vi "DecodeRobotsVSS.vi"(4 "time stamp":timestamp, 5 "offset":i32, 7 "error in (no error)":errorcluster, 8 "array w/ subset deleted in":u8[](array[numeric])) -> (0 "error out":errorcluster, 1 "array w/ subset deleted out":u8[](array[numeric]), 3 "Array":T1[](array[typedef]) {"height" format="%+4.3f"; "pixel_y" format="%+4.3f"; "pixel_x" format="%+4.3f"; "orientation" format="%+4.3f"; "y" format="%+4.3f"; "confidence" format="%4.3f"; "x" format="%+4.3f"})   [LabVIEW 2017]
uses:
  SSL Detection Robot.ctl
  <vilib>/Analysis/Matrix/Datatypes/RealMatrix.ctl
  <vilib>/Analysis/Matrix/NI_Matrix.lvlib
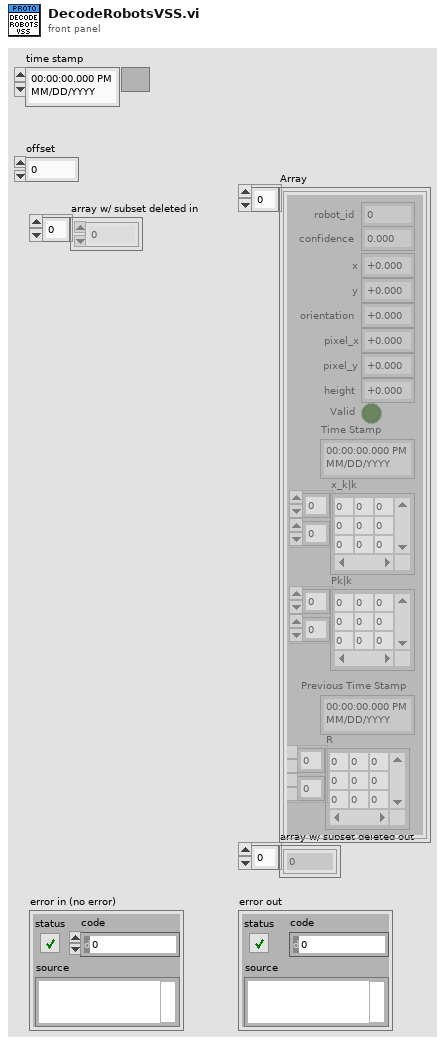
[diagram p1: front panel]
types:
  T1 = typedef "SSL Detection Robot.ctl" = cluster{"x":sgl, "robot_id":u32, "confidence":sgl, "y":sgl, "orientation":sgl, "pixel_x":sgl, "pixel_y":sgl, "height":sgl, "Valid":bool, "Time Stamp":timestamp, "x_k|k":T2, "Pk|k":T2, "Previous Time Stamp":timestamp, "R":T2}
  T2 = typedef "NI_Matrix.lvlib/RealMatrix.ctl" = dbl[][]
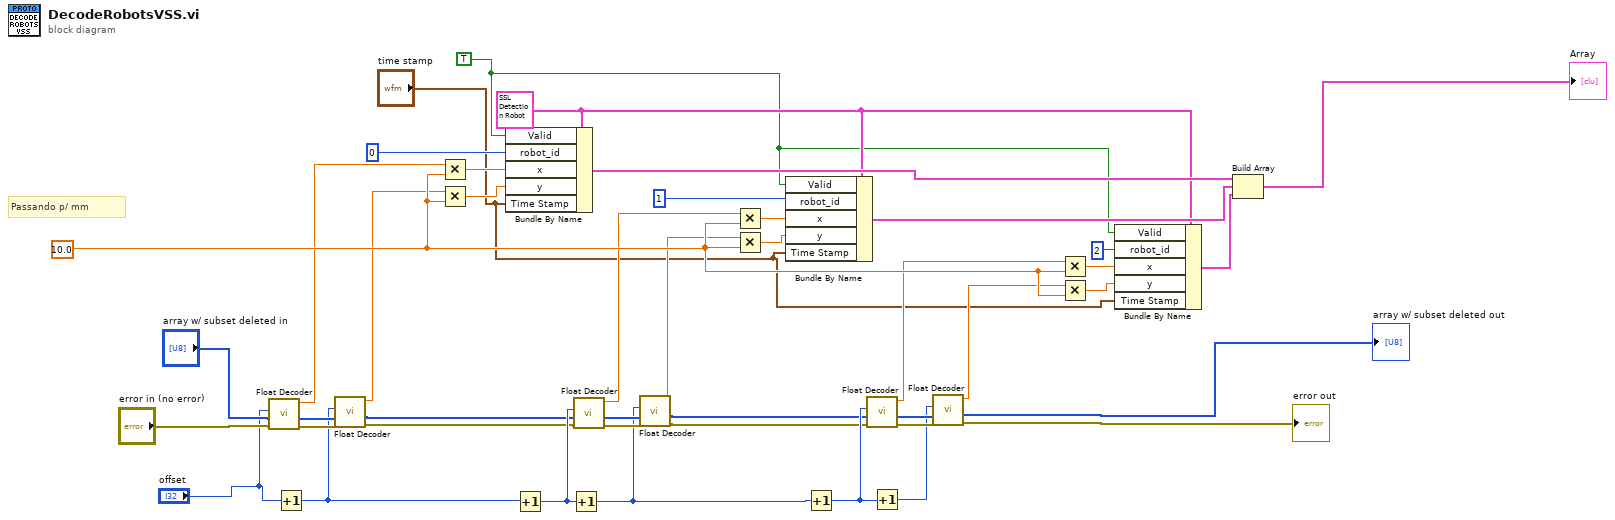
[diagram p0: block diagram]
diagram:
  w1 = TRUE
  w15 = 10.0 ("y")
  w39 = T1 {"x"=0.0, "robot_id"=0, "confidence"=0.0, "y"=0.0, "orientation"=0.0, "pixel_x"=0.0, "pixel_y"=0.0, "height"=0.0, "Valid"=FALSE, "Time Stamp"=timestamp(0 s since 1904-01-01), "x_k|k"=[], "Pk|k"=[], "Previous Time Stamp"=timestamp(0 s since 1904-01-01), "R"=[]} ("element")
  # "Passando p/ mm"
  n1 = call "Float Decoder.vi"("error in (no error)"="error in (no error)", "Array"="array w/ subset deleted in", "Key"="offset") -> ("error out"=w32:errorcluster, "array w/ subset deleted"=w31:u8[], "Float"=w14:sgl)  [unwired: 5 in, 1 out]
  n2 = Increment(x="offset") -> (x+1=w20:i32)
  n3 = call "Float Decoder.vi"("error in (no error)"=w32, "Array"=w31, "Key"=w20) -> ("error out"=w22:errorcluster, "array w/ subset deleted"=w23:u8[], "Float"=w12:sgl)  [unwired: 5 in, 1 out]
  n4 = Multiply(x=w14, y=w15) -> (x*y=w13:dbl)
  n5 = Multiply(x=w12, y=w15) -> (x*y=w11:dbl)
  n6 = Bundle By Name(cluster=w39, "Valid"=w1, "robot_id"=u32 0, "x"=w13, "y"=w11, "Time Stamp"="time stamp") -> (w42:T1)
  n7 = Increment(x=w20) -> (x+1=w27:i32)
  n8 = Increment(x=w27) -> (x+1=w21:i32)
  n9 = call "Float Decoder.vi"("error in (no error)"=w22, "Array"=w23, "Key"=w27) -> ("error out"=w33:errorcluster, "array w/ subset deleted"=w34:u8[], "Float"=w10:sgl)  [unwired: 5 in, 1 out]
  n10 = call "Float Decoder.vi"("error in (no error)"=w33, "Array"=w34, "Key"=w21) -> ("error out"=w18:errorcluster, "array w/ subset deleted"=w19:u8[], "Float"=w8:sgl)  [unwired: 5 in, 1 out]
  n11 = Multiply(x=w10, y=w15) -> (x*y=w9:dbl)
  n12 = Multiply(x=w8, y=w15) -> (x*y=w7:dbl)
  n13 = Bundle By Name(cluster=w39, "Valid"=w1, "robot_id"=u32 1, "x"=w9, "y"=w7, "Time Stamp"="time stamp") -> (w41:T1)
  n14 = Increment(x=w21) -> (x+1=w26:i32)
  n15 = call "Float Decoder.vi"("error in (no error)"=w18, "Array"=w19, "Key"=w26) -> ("error out"=w38:errorcluster, "array w/ subset deleted"=w37:u8[], "Float"=w6:sgl)  [unwired: 5 in, 1 out]
  n16 = Increment(x=w26) -> (x+1=w25:i32)
  n17 = call "Float Decoder.vi"("error in (no error)"=w38, "Array"=w37, "Key"=w25) -> ("error out"=→"error out":errorcluster, "array w/ subset deleted"=→"array w/ subset deleted out":u8[], "Float"=w4:sgl)  [unwired: 5 in, 1 out]
  n18 = Multiply(x=w6, y=w15) -> (x*y=w5:dbl)
  n19 = Multiply(x=w4, y=w15) -> (x*y=w3:dbl)
  n20 = Bundle By Name(cluster=w39, "Valid"=w1, "robot_id"=u32 2, "x"=w5, "y"=w3, "Time Stamp"="time stamp") -> (w40:T1)
  n21 = Build Array(w42, w41, w40) -> (→"Array":T1[])
